vi "Stand Alone Temp.vi"() -> ()   [LabVIEW 2009, in "Magnet.lvclass"]
uses:
  Magnet.lvclass
  Global/Sound Files.vi
panel:
  in  "warnON":bool caption="Warn On"
  in  "greater":bool caption="Temp Greater?"
  in  "warn":dbl caption="Warn at"
  out "nv%":dbl(slide) caption="NV" scale=0.0..100.0
  out "heater%":dbl(slide) caption="Heater" scale=0.0..100.0
  out "active":bool
  out "ok":bool
  in  "exit":bool
  out "temp":dbl
  # "On"
  # "K"
  # "K"
  # "Status"
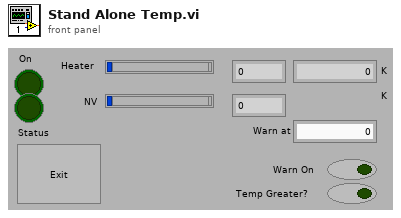
[diagram p1: front panel]
types:
  T1 = cluster{"name":string, "on?":bool, "abbrev":string}[]
  T2 = cluster{"magarray[0]":cluster{"name":string, "on?":bool, "abbrev":string}, "magarray[1]":cluster{"name":string, "on?":bool, "abbrev":string}, "magarray[2]":cluster{"name":string, "on?":bool, "abbrev":string}}
  T3 = cluster{"name":string, "on?":bool, "abbrev":string}
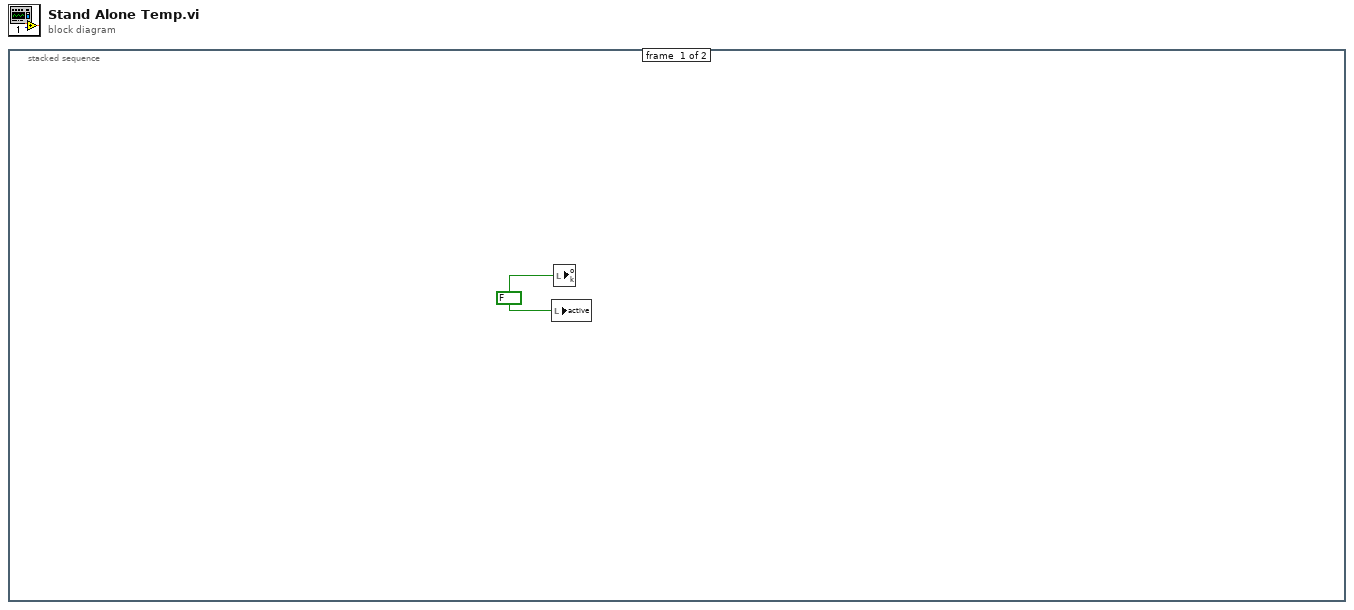
[diagram p0: block diagram]
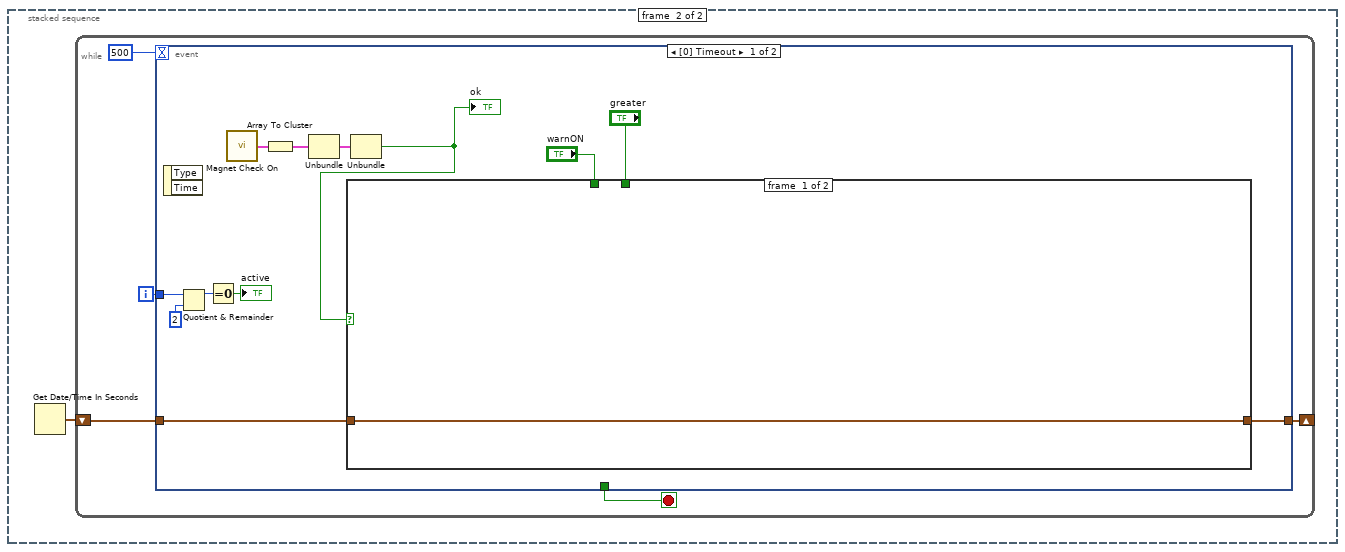
[diagram p2: hidden frame]
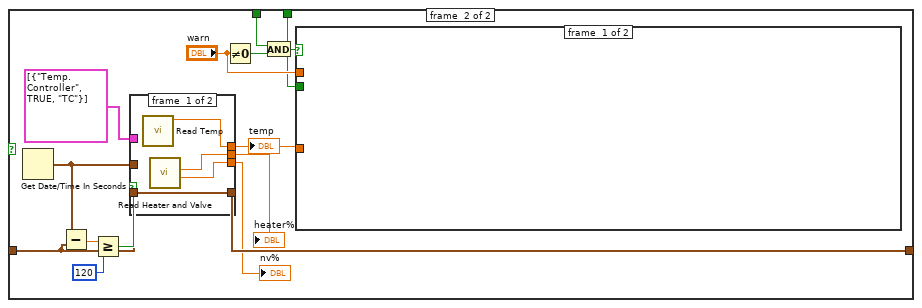
[diagram p3: hidden frame]
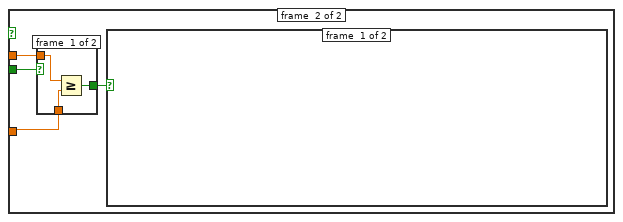
[diagram p4: hidden frame]
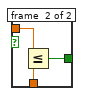
[diagram p5: hidden frame]
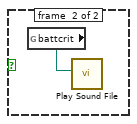
[diagram p6: hidden frame]
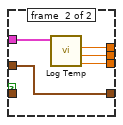
[diagram p7: hidden frame]
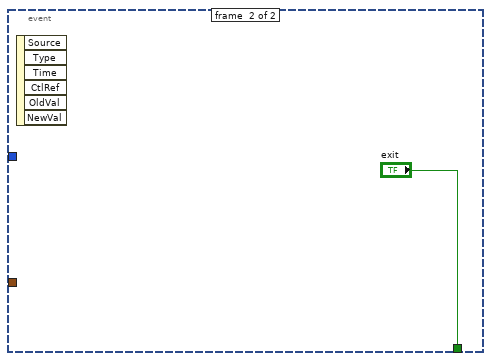
[diagram p8: hidden frame]
diagram:
  n1 = stacked-sequence {
    frame #0 {
      w1 = FALSE
      n2 = local write "active"(w1) -> ()
      n3 = local write "ok"(w1) -> ()
    }
    frame #1 {
      n4 = Get Date/Time In Seconds() -> (seconds since 1Jan1904=w2:timestamp)
      n5 = while {
        shift-right: [w3] -> _
        shift-left: w2 -> [w4]
        i -> [w5]
        stop <- w7 stop-if-true
        n6 = event shown="[0] Timeout" {
          selector: _ -> [_ _]
          dyn-events: _ -> [_ _]
          timeout: 500 -> [_ _]
          tunnel: [_ "exit"] -> w7
          tunnel: w5 -> [w19 _]
          tunnel: w4 -> [w15 _]
          tunnel: [w14 _] -> w3
          event #0 {
            n7 = event-data() -> ()  [unwired: 3 out]
            n8 = Quotient & Remainder(x=w19, y=2) -> (x-y*floor(x/y)=w17:i32)  [unwired: 1 out]
            n9 = Equal To 0?(x=w17) -> (x = 0?=→"active":bool)
            n10 = call "Magnet Check On.vi"() -> ("magarray"=w13:T1)  [unwired: 5 out]
            n11 = Array To Cluster(array=w13) -> (cluster=w12:T2)
            n12 = Unbundle(w12) -> ("magarray[1]"=w11:T3)  [unwired: 2 out]
            n13 = Unbundle(w11) -> ("on?"=w10:bool)  [unwired: 2 out]
            "ok" <- w10
            n14 = case shown="True" w10 {
              tunnel: w15 -> [w20 w30]
              tunnel: [w20 w29] -> w14
              tunnel: "greater" -> [_ w24]
              tunnel: "warnON" -> [_ w21]
              frame #0 {
              }
              frame #1 {
                n15 = Get Date/Time In Seconds() -> (seconds since 1Jan1904=w31:timestamp)
                n16 = Subtract(x=w31, y=w30) -> (x-y=w35:dbl)
                n17 = Greater Or Equal?(x=w35, y=120) -> (x >= y?=w33:bool)
                n18 = case shown="False" w33 {
                  tunnel: [w50 w55] -> w25
                  tunnel: cluster{string, bool, string}[] [{"Temp. Controller", TRUE, "TC"}] -> [_ w54]
                  tunnel: w31 -> [_ w53]
                  tunnel: w30 -> [w49 _]
                  tunnel: [w49 w53] -> w29
                  tunnel: [w47 w52] -> w28
                  tunnel: [w48 w51] -> w27
                  frame #0 {
                    n19 = call "Read Temp.vi"() -> ("temp"=w50:dbl)  [unwired: 7 out]
                    n20 = call "Read Heater and Valve.vi"() -> ("valve%"=w48:dbl, "heater%"=w47:dbl)  [unwired: 10 out]
                  }
                  frame #1 {
                    n21 = call "Log Temp.vi"("magarray"=w54) -> ("valve%"=w51:dbl, "heater%"=w52:dbl, "temp"=w55:dbl)  [unwired: 8 out]
                  }
                }
                "temp" <- w25
                "heater%" <- w28
                "nv%" <- w27
                n22 = Not Equal To 0?(x="warn") -> (x != 0?=w22:bool)
                n23 = And(x=w21, y=w22) -> (x .and. y?=w23:bool)
                n24 = case shown="True" w23 {
                  tunnel: "warn" -> [_ w39]
                  tunnel: w25 -> [_ w38]
                  tunnel: w24 -> [_ w36]
                  frame #0 {
                  }
                  frame #1 {
                    n25 = case shown="True" w36 {
                      tunnel: w39 -> [w40 w45]
                      tunnel: w38 -> [w41 w44]
                      tunnel: [w42 w43] -> w37
                      frame #0 {
                        n26 = Greater Or Equal?(x=w40, y=w41) -> (x >= y?=w42:bool)
                      }
                      frame #1 {
                        n27 = Less Or Equal?(x=w45, y=w44) -> (x <= y?=w43:bool)
                      }
                    }
                    n28 = case shown="True" w37 {
                      frame #0 {
                      }
                      frame #1 {
                        n29 = global read "Sound Files.vi" "battcrit"() -> (w46:path)
                        n30 = call <vilib>:"Play Sound File.vi"("path"=w46) -> ()  [unwired: 3 in, 8 out]
                      }
                    }
                  }
                }
              }
            }
          }
          event #1 {
            n31 = event-data() -> ()  [unwired: 7 out]
          }
        }
      }
    }
  }
